vi "Control Shooter.vi"(11 "Avoid Race Condition":bool) -> ()   [LabVIEW 2020]
uses:
  Framework/Robot Global Data.vi
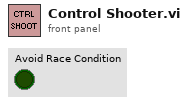
[diagram p1: front panel]
types:
  T1 = typedef "Command Status Info.ctl" = cluster{"Name":string, "Status":T2, "notifier out":T3}
  T2 = typedef "Completion Status.ctl" = enum16{"Successful", "Aborted", "Incomplete"}
  T3 = typedef "Completion Notifier.ctl" = refnum<notifier>
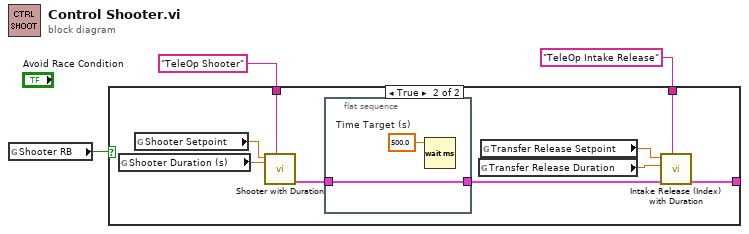
[diagram p0: block diagram]
diagram:
  n1 = global read "Robot Global Data.vi" "Shooter RB"() -> (w1:bool)
  n2 = case shown="True" w1 {
    tunnel: [_ w6] -> _
    tunnel: "TeleOp Intake Release" ("Description") -> [_ w5]
    tunnel: "TeleOp Shooter" ("Description") -> [_ w4]
    frame False {
    }
    frame True {
      n3 = global read "Robot Global Data.vi" "Shooter Duration (s)"() -> (w10:dbl)
      n4 = global read "Robot Global Data.vi" "Shooter Setpoint"() -> (w9:dbl)
      n5 = call "Shooter with Duration .vi"("Description"=w4, "Duration (s)"=w10, "Setpoint"=w9) -> ("Command Info Out"=w8:T1)  [unwired: 8 in]
      n6 = flat-sequence {
        tunnel: w8 -> [w14]
        tunnel: [w14] -> w7
        frame #0 {
          w13 = 500.0  # Time Target (s)
          n7 = Wait (ms)(milliseconds to wait=w13) -> ()  [unwired: 1 out]
        }
      }
      n8 = global read "Robot Global Data.vi" "Transfer Release Duration"() -> (w11:dbl)
      n9 = global read "Robot Global Data.vi" "Transfer Release Setpoint"() -> (w12:dbl)
      n10 = call "Intake Release (Index) with Duration.vi"("Description"=w5, "Command Info In"=w7, "Duration (s)"=w11, "Setpoint"=w12) -> ("Command Info Out"=w6:T1)  [unwired: 7 in]
    }
  }
